vi "PostPersonnel.vi"(7 "LabVIEW Web Service Request":refnum<class "Web Request.lvclass">, 9 "Data":string, 10 "Command":string, 11 "UID":string) -> (2 "Response":string)   [LabVIEW 2015]
uses:
  <vilib>/wsapi/Web Request.lvclass
  TypeDef/PersonnelActions.ctl
  TypeDef/RoomsActionEnum.ctl
  TypeDef/RequestActionEnum.ctl
  LVClasses/Personnel/Personnel.lvclass/Personnel.ctl
  LVClasses/Request/Request.lvclass/Request.ctl
  LVClasses/Request/Read Request Type.vi
  LVClasses/Request/Read PersonnelType.vi
  LVClasses/Request/Read StartName.vi
  LVClasses/Request/Read PUID.vi
  LVClasses/Request/Read Summary.vi
  LVClasses/Personnel/Read UniqueID.vi
  LVClasses/Personnel/Read Role.vi
  LVClasses/Request/Request.lvclass
  LVClasses/Personnel/Personnel.lvclass
panel:
  out "output array":string[](array[string])
  in  "s":bool
  out "current time":timestamp
  out "postdata":string
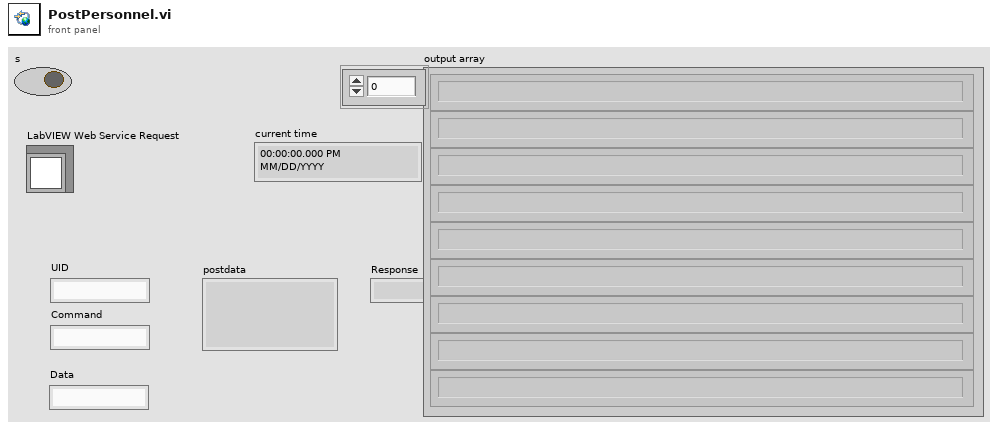
[diagram p1: front panel]
types:
  T1 = typedef "PersonnelActions.ctl" = enum16{"Init", "Read Personnel", "Add Personnel", "Remove Personnel", "Read Name", "Write Name", "Read Role", "Write Role", "Read Requests", "Add Requests", "Remove Requests", "Read PUIDs", "Read PUIDs for Role"}
  T2 = typedef "RequestActionEnum.ctl" = enum16{"Init", "ReadRequests", "ReadRequest", "AddRequest", "RemoveRequest", "ToDisk", "Ack", "Complete", "CheckAlarms", "PIntoRoom", "Read Summary", "GetRequestForRoom"}
  T3 = typedef "RoomsActionEnum.ctl" = enum16{"Init", "Add Room", "Remove Room", "Read Room", "Read Flag", "Read Flag State", "Write Flag State", "Read Flag Color", "Write Flag Color", "Read Bed Vacant", "Write Bed Vacant", "Read Personnel", "Add Personnel", "Remove Personnel", "Read Requests", "Add Request", "Remove Request", "Read Beacon ID", "Write Beacon ID", "Write Bed URL", "Read Bed URL", "Read Rooms Numbers", "Write Flag"}
  T4 = typedef "Personnel.lvclass/PersonnelType.ctl" = enum16{"Nurse", "Doctor", "Cleanning", "Admin"}
  T5 = typedef "Request.lvclass/RequestType.ctl" = enum16{"Specific Call To Room", "General Call To Room"}
  T6 = typedef "Request.lvclass/PersonnelType.ctl" = u16
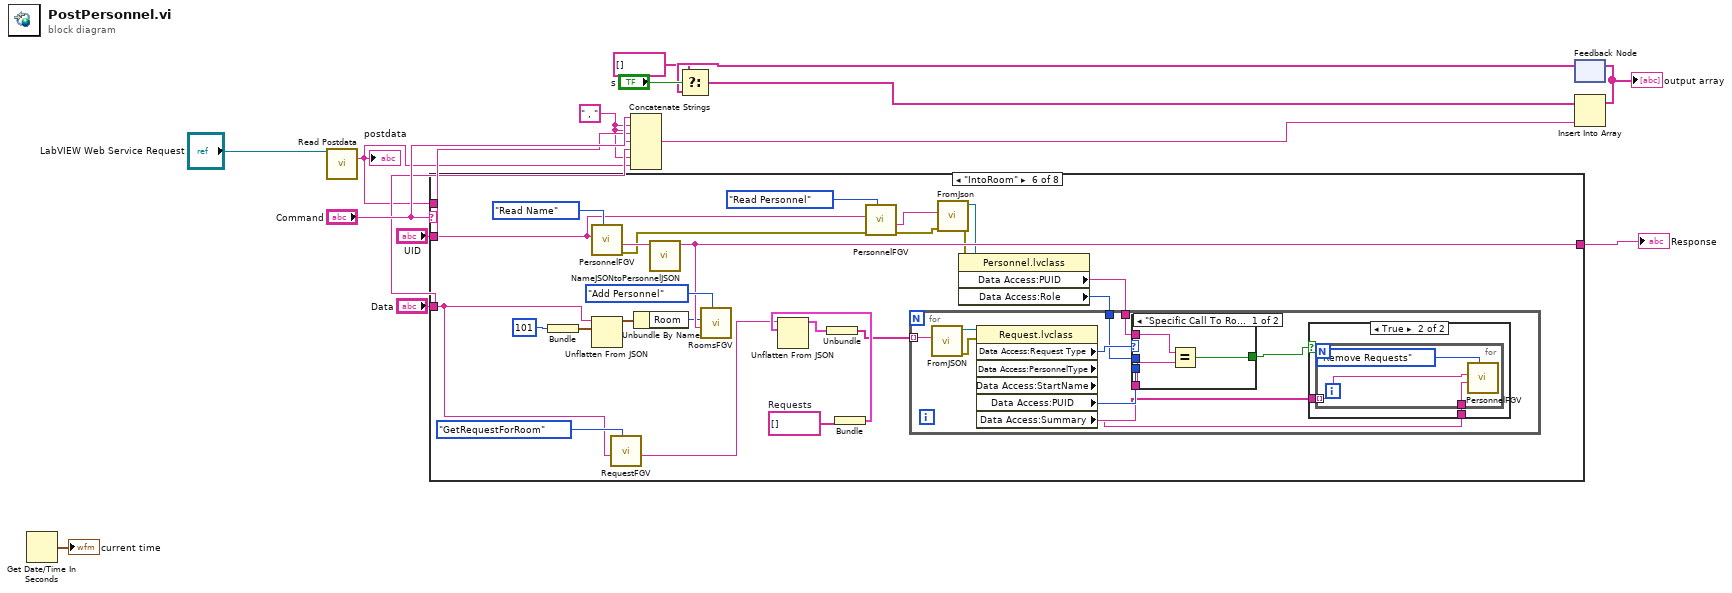
[diagram p0: block diagram]
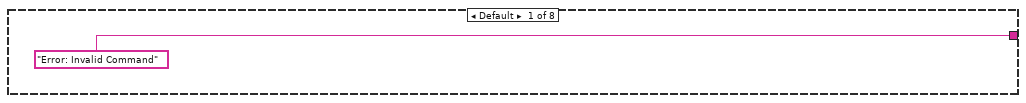
[diagram p2: hidden frame]
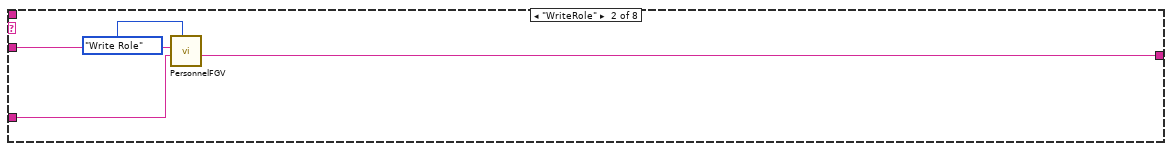
[diagram p3: hidden frame]
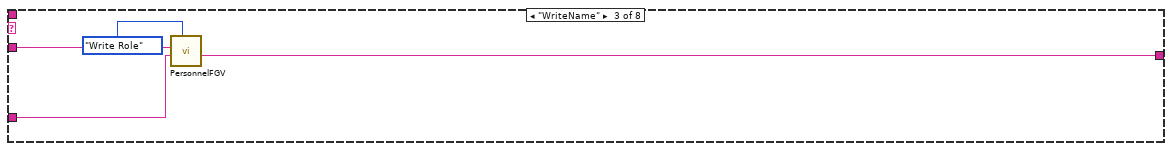
[diagram p4: hidden frame]
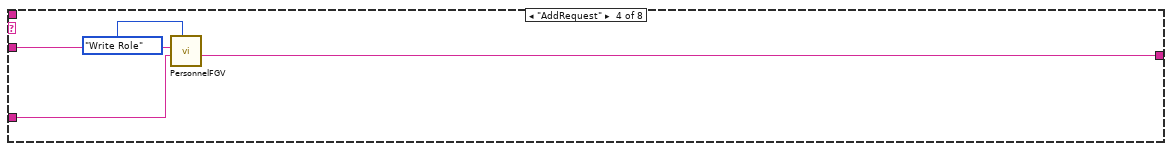
[diagram p5: hidden frame]
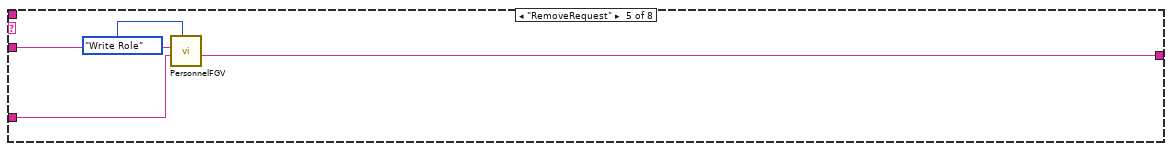
[diagram p6: hidden frame]
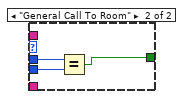
[diagram p8: hidden frame]
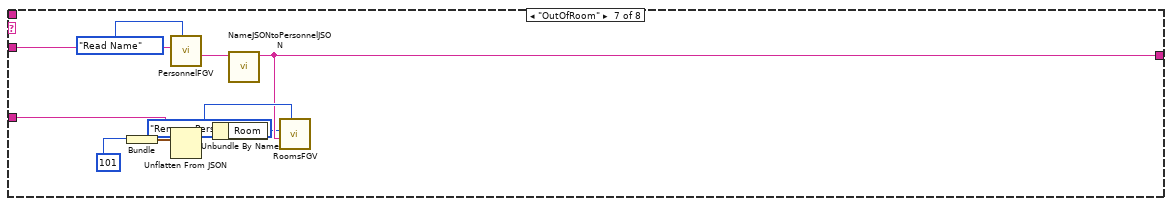
[diagram p9: hidden frame]
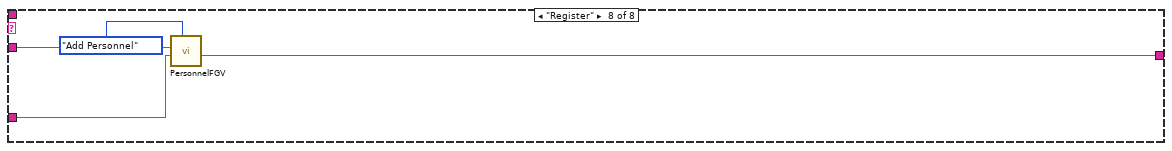
[diagram p10: hidden frame]
diagram:
  w1 = " , " ("string")
  n1 = Get Date/Time In Seconds() -> (seconds since 1Jan1904=→"current time":timestamp)
  n2 = call <vilib>:"Read Postdata.vi"("LabVIEW Web Service Request"="LabVIEW Web Service Request") -> ("postdata"=w8:string)  [unwired: 12 in, 2 out]
  "postdata" <- w8
  n3 = case shown="\"IntoRoom\"" "Command" {
    tunnel: w8 -> [_ _ _ _ _ _ _ _]
    tunnel: "UID" -> [_ w18 w22 w26 w30 w38 w86 w90]
    tunnel: "Data" -> [_ w17 w21 w25 w29 w46 w83 w89]
    tunnel: ["Error: Invalid Command" ("Data Out") w16 w20 w24 w28 w49 w80 w88] -> w13
    frame Default {
    }
    frame "WriteRole" {
      n4 = call "PersonnelFGV.vi"("Actions"=PersonnelActions."Write Role", "Data In"=w17, "PUID"=w18) -> ("Data Out"=w16:string)  [unwired: 7 in, 1 out]
    }
    frame "WriteName" {
      n5 = call "PersonnelFGV.vi"("Actions"=PersonnelActions."Write Role", "Data In"=w21, "PUID"=w22) -> ("Data Out"=w20:string)  [unwired: 7 in, 1 out]
    }
    frame "AddRequest" {
      n6 = call "PersonnelFGV.vi"("Actions"=PersonnelActions."Write Role", "Data In"=w25, "PUID"=w26) -> ("Data Out"=w24:string)  [unwired: 7 in, 1 out]
    }
    frame "RemoveRequest" {
      n7 = call "PersonnelFGV.vi"("Actions"=PersonnelActions."Write Role", "Data In"=w29, "PUID"=w30) -> ("Data Out"=w28:string)  [unwired: 7 in, 1 out]
    }
    frame "IntoRoom" {
      w45 = string[] []  # Requests
      n8 = Bundle("Room"=101) -> (w52:cluster{"Room":i32})  [unwired: 1 in]
      n9 = call "PersonnelFGV.vi"("Actions"=PersonnelActions."Read Name", "PUID"=w38) -> ("error out"=w40:errorcluster, "Data Out"=w50:string)  [unwired: 8 in]
      n10 = Unflatten From JSON(JSON string=w46, type and defaults=w52) -> (value=w51:cluster{"Room":i32})  [unwired: 5 in, 1 out]
      n11 = call "RequestFGV.vi"("Actions"=RequestActionEnum."GetRequestForRoom", "Data In"=w46) -> ("Data Out"=w41:string)  [unwired: 8 in, 1 out]
      n12 = Unbundle By Name(w51) -> ("Room"=w48:i32)
      n13 = call "NameJSONtoPersonnelJSON.vi"("Name JSON"=w50) -> ("Personnel JSON"=w49:string)  [unwired: 10 in]
      n14 = call "RoomsFGV.vi"("Actions"=RoomsActionEnum."Add Personnel", "Data In"=w49, "Room"=w48) -> ()  [unwired: 7 in, 2 out]
      n15 = Bundle("Requests"=w45) -> (w44:cluster{"Requests":string[]})  [unwired: 1 in]
      n16 = Unflatten From JSON(JSON string=w41, type and defaults=w44) -> (value=w43:cluster{"Requests":string[]})  [unwired: 5 in, 1 out]
      n17 = Unbundle(w43) -> ("Requests"=w42:string[])
      n18 = call "PersonnelFGV.vi"("Actions"=PersonnelActions."Read Personnel", "error in (no error)"=w40, "PUID"=w38) -> ("error out"=w34:errorcluster, "Data Out"=w37:string)  [unwired: 7 in]
      n19 = call "FromJson.vi"("error in (no error)"=w34, "PersonnelJson"=w37) -> ("error out"=w35:errorcluster, "Personnel out"=w36:refnum<class "Personnel.lvclass">)  [unwired: 8 in]
      n20 = property class="Personnel.lvclass"(reference=w36, error in=w35) -> ("Data Access:PUID"=w33:string, "Data Access:Role"=w32:T4)  [unwired: 2 out]
      n21 = for {
        tunnel: w42 -> [w66] mode=indexing
        tunnel: w33 -> [w61]
        tunnel: w32 -> [w62]
        n22 = call "FromJSON.vi"("Request"=w66) -> ("error out"=w65:errorcluster, "Request out"=w59:refnum<class "Request.lvclass">)  [unwired: 9 in]
        n23 = property class="Request.lvclass"(reference=w59, error in=w65) -> ("Data Access:Request Type"=w64:T5, "Data Access:PersonnelType"=w63:T6, "Data Access:StartName"=w60:string, "Data Access:PUID"=w57:string[], "Data Access:Summary"=w56:string)  [unwired: 2 out]
        n24 = case shown="\"Specific Call To Room\", Default" w64 {
          tunnel: w63 -> [_ w76]
          tunnel: w62 -> [_ w77]
          tunnel: [w72 w75] -> w58
          tunnel: w61 -> [w74 _]
          tunnel: w60 -> [w73 _]
          frame "Specific Call To Room", Default {
            n25 = Equal?(x=w74, y=w73) -> (x = y?=w72:bool)
          }
          frame "General Call To Room" {
            n26 = Equal?(x=w77, y=w76) -> (x = y?=w75:bool)
          }
        }
        n27 = case shown="True" w58 {
          tunnel: w57 -> [_ w68]
          tunnel: w56 -> [_ w67]
          frame False {
          }
          frame True {
            n28 = for {
              tunnel: w68 -> [w70] mode=indexing
              tunnel: w67 -> [w69]
              n29 = call "PersonnelFGV.vi"("Actions"=PersonnelActions."Remove Requests", "Data In"=w69, "PUID"=w70) -> ()  [unwired: 7 in, 2 out]
            }
          }
        }
      }
    }
    frame "OutOfRoom" {
      n30 = Bundle("Room"=101) -> (w84:cluster{"Room":i32})  [unwired: 1 in]
      n31 = call "PersonnelFGV.vi"("Actions"=PersonnelActions."Read Name", "PUID"=w86) -> ("Data Out"=w81:string)  [unwired: 8 in, 1 out]
      n32 = Unflatten From JSON(JSON string=w83, type and defaults=w84) -> (value=w82:cluster{"Room":i32})  [unwired: 5 in, 1 out]
      n33 = Unbundle By Name(w82) -> ("Room"=w78:i32)
      n34 = call "NameJSONtoPersonnelJSON.vi"("Name JSON"=w81) -> ("Personnel JSON"=w80:string)  [unwired: 10 in]
      n35 = call "RoomsFGV.vi"("Actions"=RoomsActionEnum."Remove Personnel", "Data In"=w80, "Room"=w78) -> ()  [unwired: 7 in, 2 out]
    }
    frame "Register" {
      n36 = call "PersonnelFGV.vi"("Actions"=PersonnelActions."Add Personnel", "Data In"=w89, "PUID"=w90) -> ("Data Out"=w88:string)  [unwired: 7 in, 1 out]
    }
  }
  "Response" <- w13
  n37 = Concatenate Strings("Command", w1, "UID", w1, "Data", w1, w8) -> (w7:string)
  n38 = feedback #1() -> (w4:string[])  [unwired: 1 in]
  n39 = Select(t=string[] [], s="s", f=w4) -> (s? t:f=w2:string[])
  n40 = Insert Into Array(array=w2, new element=w7) -> (w6:string[])  [unwired: 1 in]
  "output array" <- w6
  n41 = feedback-in #1(w6) -> ()
